vi "UART_B_(SubVI).vi"(0 "Señal_1 in":dbl, 1 "Señal_2 in":dbl, 2 "Señal_3 in":dbl, 3 "Señal 6":dbl, 4 "Señal 7":dbl) -> (7 "US_3 6":string, 8 "Trama de envio 2":string, 9 "US_3 5":string, 10 "US_1 2":string, 11 "Sensor 7":dbl, 12 "US_2 2":string, 13 "Sensor 6":dbl, 14 "Sensor_1 2":dbl, 15 "Sensor_2 2":dbl, 16 "Trama Recibida 2":string, 17 "Sensor_3 2":dbl, 18 "US_3 4":string)   [LabVIEW 2019]
uses:
  <vilib>/myRIO/Instrument Drivers/Onboard IO/UART/typedef/VISA Configuration.ctl
  <vilib>/Instr/_visa.llb/VISA Configure Serial Port (Instr).vi
  <vilib>/myRIO/Express VI/Onboard IO/UART/UART Express VI.xnode
  <vilib>/myRIO/Instrument Drivers/Onboard IO/UART/UART.lvlib
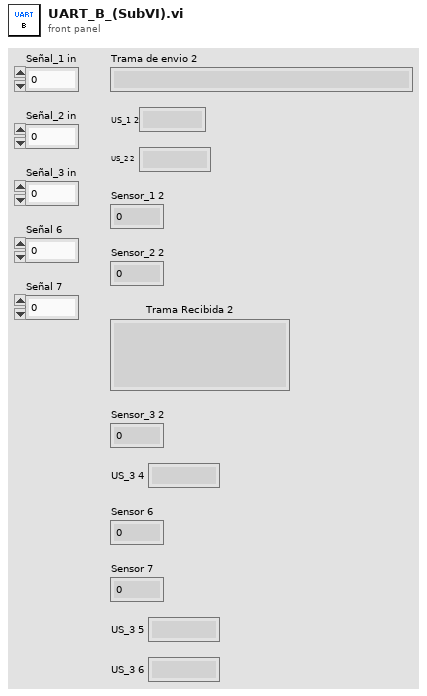
[diagram p1: front panel]
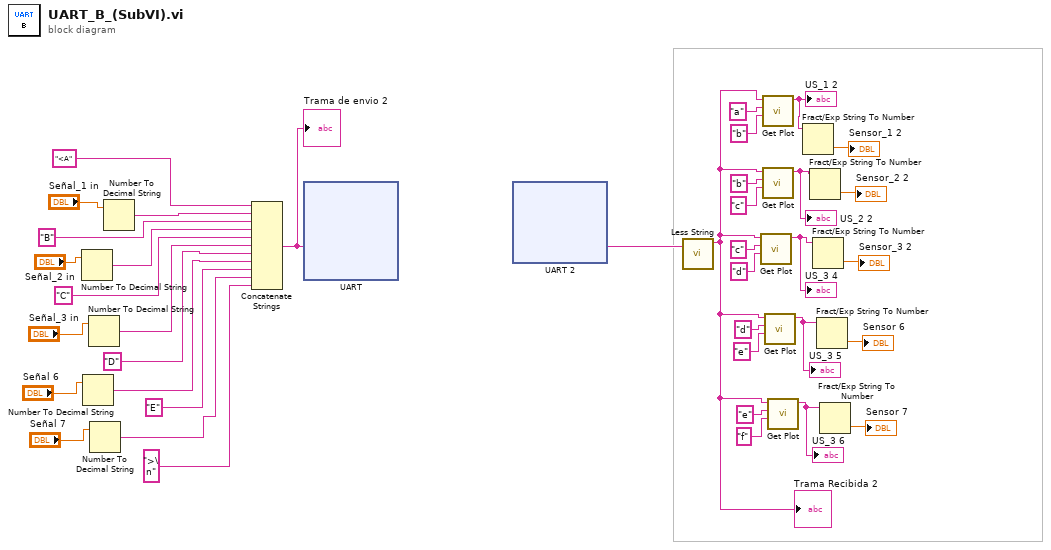
[diagram p0: block diagram]
diagram:
  n1 = Number To Decimal String(number="Señal_2 in") -> (decimal integer string=w24:string)  [unwired: 1 in]
  n2 = Number To Decimal String(number="Señal 6") -> (decimal integer string=w13:string)  [unwired: 1 in]
  n3 = Number To Decimal String(number="Señal_3 in") -> (decimal integer string=w22:string)  [unwired: 1 in]
  n4 = Number To Decimal String(number="Señal 7") -> (decimal integer string=w11:string)  [unwired: 1 in]
  n5 = Number To Decimal String(number="Señal_1 in") -> (decimal integer string=w26:string)  [unwired: 1 in]
  n6 = Concatenate Strings("<A" ("string"), w26, "B" ("string"), w24, "C" ("string"), w22, "D" ("string"), w13, "E" ("string"), w11, ">\n" ("string")) -> (w17:string)
  "Trama de envio 2" <- w17
  n7 = xnode "UART"("Characters to Write"=w17) -> ()  [unwired: 1 in, 2 out]
  n8 = xnode "UART 2"() -> ("Characters Read"=w27:string)  [unwired: 1 in, 1 out]
  n9 = call "Less String.vi"("Input String"=w27) -> ("Out String"=w1:string)  [unwired: 10 in]
  "Trama Recibida 2" <- w1
  n10 = call "Get Plot.vi"("Stop"="d", "Start"="c", "Input String"=w1) -> ("Out String"=w28:string)  [unwired: 8 in]
  "US_3 4" <- w28
  n11 = call "Get Plot.vi"("Stop"="b", "Start"="a", "Input String"=w1) -> ("Out String"=w33:string)  [unwired: 8 in]
  "US_1 2" <- w33
  n12 = call "Get Plot.vi"("Stop"="c", "Start"="b", "Input String"=w1) -> ("Out String"=w29:string)  [unwired: 8 in]
  "US_2 2" <- w29
  n13 = call "Get Plot.vi"("Stop"="e", "Start"="d", "Input String"=w1) -> ("Out String"=w6:string)  [unwired: 8 in]
  "US_3 5" <- w6
  n14 = call "Get Plot.vi"("Stop"="f", "Start"="e", "Input String"=w1) -> ("Out String"=w2:string)  [unwired: 8 in]
  "US_3 6" <- w2
  n15 = Fract/Exp String To Number(string=w33) -> (number=→"Sensor_1 2":dbl)  [unwired: 3 in, 1 out]
  n16 = Fract/Exp String To Number(string=w29) -> (number=→"Sensor_2 2":dbl)  [unwired: 3 in, 1 out]
  n17 = Fract/Exp String To Number(string=w28) -> (number=→"Sensor_3 2":dbl)  [unwired: 3 in, 1 out]
  n18 = Fract/Exp String To Number(string=w6) -> (number=→"Sensor 6":dbl)  [unwired: 3 in, 1 out]
  n19 = Fract/Exp String To Number(string=w2) -> (number=→"Sensor 7":dbl)  [unwired: 3 in, 1 out]
